vi "Get Domain.vi"(8 "error in (no error)":errorcluster, 11 "Domain_Evolut_2D_Rect in":refnum<class "NI_Domain_Evolut_2D_Rect.lvclass">) -> (0 "error out":errorcluster, 2 "domain":variant, 3 "Domain_Evolut_2D_Rect out":refnum<class "NI_Domain_Evolut_2D_Rect.lvclass">)   [LabVIEW 2017, in "NI_PDE.lvlib" / "NI_Domain_Evolut_2D_Rect.lvclass"]
uses:
  <vilib>/gmath/pde.llb/DomainClass/Domain_Evolut_2D_Rect/NI_Domain_Evolut_2D_Rect.lvclass
  <vilib>/gmath/pde.llb/DomainClass/Domain_Evolut_2D_Rect/Domain Data.ctl
  <vilib>/gmath/pde.llb/DomainClass/Domain_Evolut_2D_Rect/NI_Domain_Evolut_2D_Rect.lvclass/NI_Domain_Evolut_2D_Rect.ctl
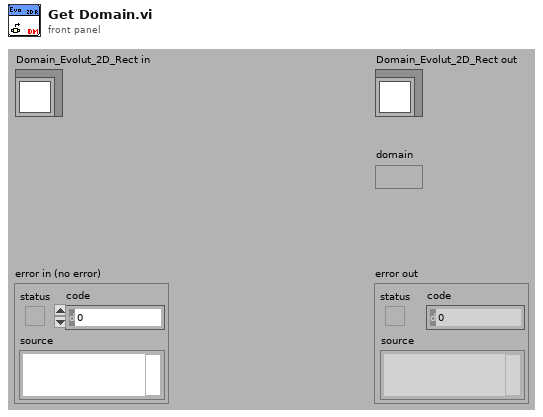
[diagram p1: front panel]
types:
  T1 = typedef "NI_PDE.lvlib/NI_Domain_Evolut_2D_Rect.lvclass/Domain Data.ctl" = cluster{"T":cluster{"initial t":dbl, "final t":dbl, "# of t-points":i32}, "X":cluster{"start x":dbl, "end x":dbl, "# of x-points":i32}, "Y":cluster{"start y":dbl, "end y":dbl, "# of y-points":i32}}
  T2 = cluster{"initial t":dbl, "final t":dbl, "# of t-points":i32}
  T3 = cluster{"start x":dbl, "end x":dbl, "# of x-points":i32}
  T4 = cluster{"start y":dbl, "end y":dbl, "# of y-points":i32}
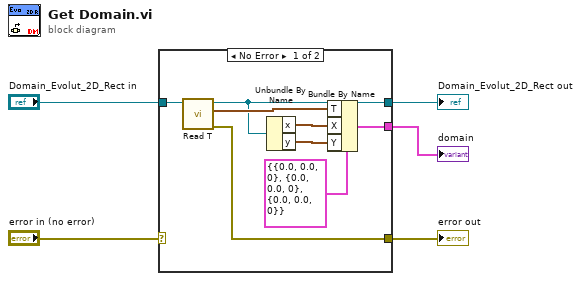
[diagram p0: block diagram]
diagram:
  n1 = case shown="No Error" "error in (no error)" {
    selector: "error in (no error)" -> [_ w15]
    tunnel: "Domain_Evolut_2D_Rect in" -> [w13 w14]
    tunnel: [w8 w14] -> w5
    tunnel: [w12 w15] -> w4
    tunnel: [w9 _] -> w1
    frame No Error {
      n2 = call-dynamic "Read T.vi"("Domain_Evolut.lvclass in"=w13) -> ("error out"=w12:errorcluster, "t"=w10:T2, "Domain_Evolut.lvclass out"=w8:refnum<class "NI_Domain_Evolut_2D_Rect.lvclass">)  [unwired: 1 in, 7 out]
      n3 = Unbundle By Name(w8) -> ("x"=w7:T3, "y"=w6:T4)
      n4 = Bundle By Name(cluster=T1 {"T"={"initial t"=0.0, "final t"=0.0, "# of t-points"=0}, "X"={"start x"=0.0, "end x"=0.0, "# of x-points"=0}, "Y"={"start y"=0.0, "end y"=0.0, "# of y-points"=0}} ("domain data"), "T"=w10, "X"=w7, "Y"=w6) -> (w9:T1)
    }
    frame Error {
    }
  }
  "Domain_Evolut_2D_Rect out" <- w5
  "error out" <- w4
  "domain" <- w1
